vi "MainVI_Project3.vi"() -> ()   [LabVIEW 2025]
uses:
  <vilib>/MakerHub/LINX/Public/Peripherals/Digital/Digital Write 1 Chan.vi
  <vilib>/MakerHub/LINX/Public/Peripherals/Digital/Digital Write N Chans.vi
  <vilib>/MakerHub/LINX/Private/Local IO/LinxDigitalWrite.vi
  <vilib>/MakerHub/LINX/Public/Utilities/Check Channel.vi
  <vilib>/MakerHub/LINX/Public/Utilities/Open Serial.vi
  <vilib>/MakerHub/LINX/Private/Utilties/Generate Error.vi
  <vilib>/MakerHub/LINX/LMH-LINX.lvlib
panel:
  out "Patient's Heart Rate (BPM)":dbl format="%#_12g"
  out "Raw Signal with Smoothed Signal Waveform Graph":waveform(dbl)[](graph)
  in  "Sampling Frequency (Hz)":dbl
  in  "Sampling Duration (s)":dbl
  out "STD dt":dbl
  out "Holding Last Good HR":bool
  out "Good Signal !!":bool
  out "Full AutoCorrelation Waveform Graph":dbl[](graph)
  out "Peak Markers XY Graph":T1(graph)
  out "# Valid Peaks":i32
  in  "AutoCorrelation Peak Ratio Threshold":dbl
  in  "AutoCorrelation Max Lag":dbl
  in  "Tolerance Fraction":dbl
  out "Periodic Signal?":bool
  out "Best Lag":dbl
  out "AutoCorr Peak Amplitudes":dbl[](array[numeric])
  out "AutoCorrelation - Right Side":dbl[](array[numeric])
  out "AutoCorrelation Peak Locations":dbl[](array[numeric])
  out "Right Side AutoCorrelation Waveform Graph":dbl[](graph)
  in  "Autocorrelation Peak Width":dbl
  in  "Autocorrelation Peak Threshold":dbl
  in  "Autocorrelation Min Lag":dbl
  in  "Max Lag Index":dbl
  in  "Min Lag Index":dbl
  out "Periods (s)":dbl[](array[numeric])
  out "Filtered Lag Array":dbl[](array[numeric])
  out "Valid HR?":bool
  out "Valid Peaks Found?":bool
  out "Peak Amplitudes":dbl[](array[numeric])
  out "Peak Locations":dbl[](array[numeric])
  in  "Peak Threshold":dbl
  in  "Peak Width":dbl
  out "Sample Count":i32
  out "Raw Voltage":dbl
  out "Heart Rate Trend Waveform Chart":dbl(graph)
  out "Heart Rate (BPM)":dbl
  out "Normalized Signal Waveform Graph":waveform(dbl)(graph)
  out "Raw Signal Waveform Graph":waveform(dbl)(graph)
  out "dt (sec)":dbl
  out "Detrended Signal Waveform Graph":waveform(dbl)(graph)
  out "Smoothed Signal Waveform Graph":waveform(dbl)(graph)
  out "Error Out":errorcluster
  in  "Serial Port":refnum<visa-resource-name>="N/A"
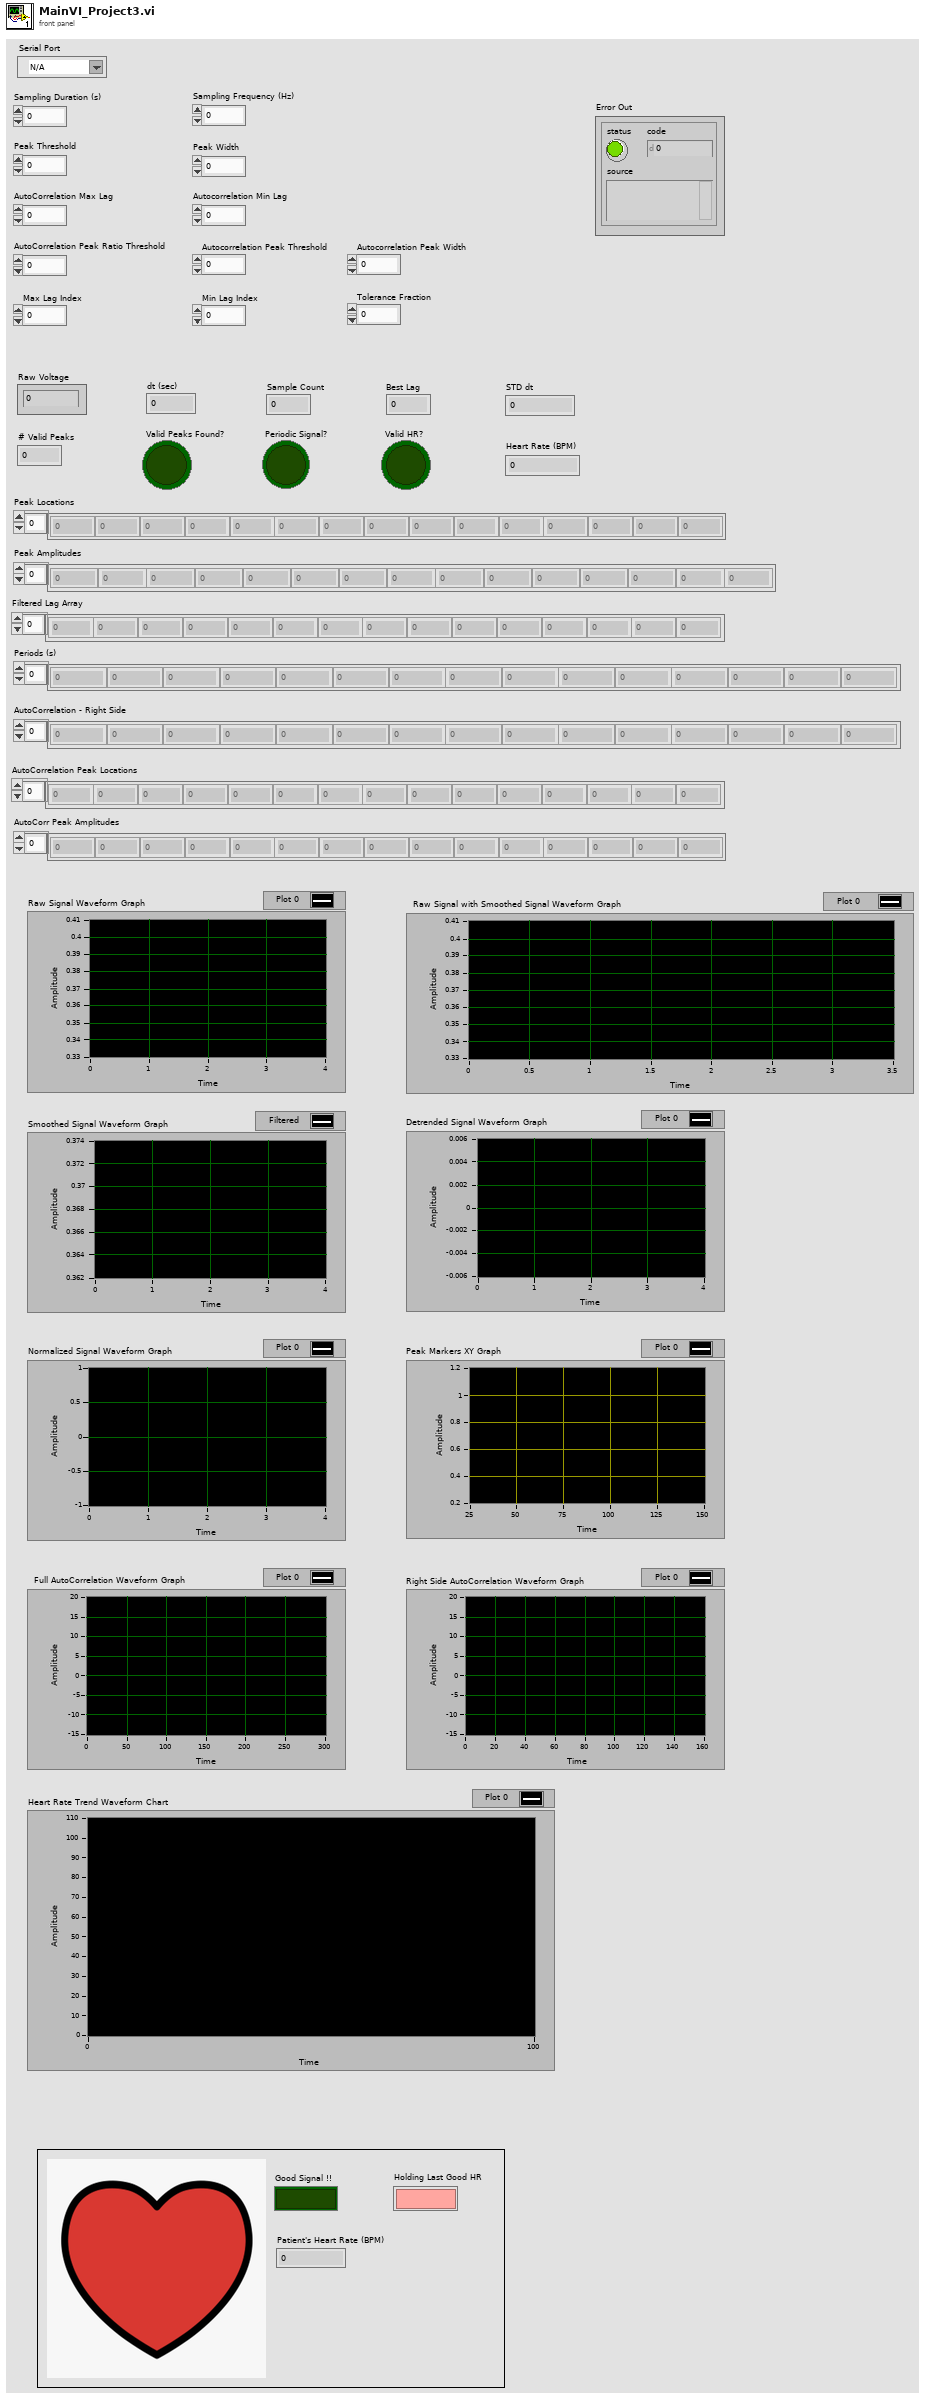
[diagram p1: front panel]
types:
  T1 = cluster{"Peak Locations":dbl[], "Peak Amplitudes":dbl[]}
  T2 = typedef "LMH-LINX.lvlib/LINX Ref.ctl" = cluster{"IO":T3, "Interface":T4, "LINX Device Config":T5}
  T3 = typedef "LMH-LINX.lvlib/Platform.ctl" = enum16{"Remote", "Local"}
  T4 = typedef "LMH-LINX.lvlib/Interface.ctl" = enum16{"Serial", "TCP"}
  T5 = typedef "LMH-LINX.lvlib/Device.lvlib/LINX Device Config.ctl" = cluster{"Interface":T4, "COM Port":refnum<visa-resource-name>, "TCP Configuration":T6, "Device Family":u8, "Device ID":u8, "Device Name":string, "TCP Ref":refnum<k5>, "Channels":T7}
  T6 = typedef "LMH-LINX.lvlib/Device.lvlib/TCP Config.ctl" = cluster{"IP Address":string, "Port":u16}
  T7 = typedef "LMH-LINX.lvlib/Channels.ctl" = cluster{"DI":u8[], "DO":u8[], "AI":u8[], "AO":u8[], "PWM":u8[], "QE":u8[], "UART":u8[], "I2C 2":u8[], "SPI":u8[], "CAN":u8[], "Servo":u8[], "AI Ref (V)":dbl, "AI Resolution (Bits)":u8, "AO Ref (V)":dbl, "AO Resolution (Bits)":u8}
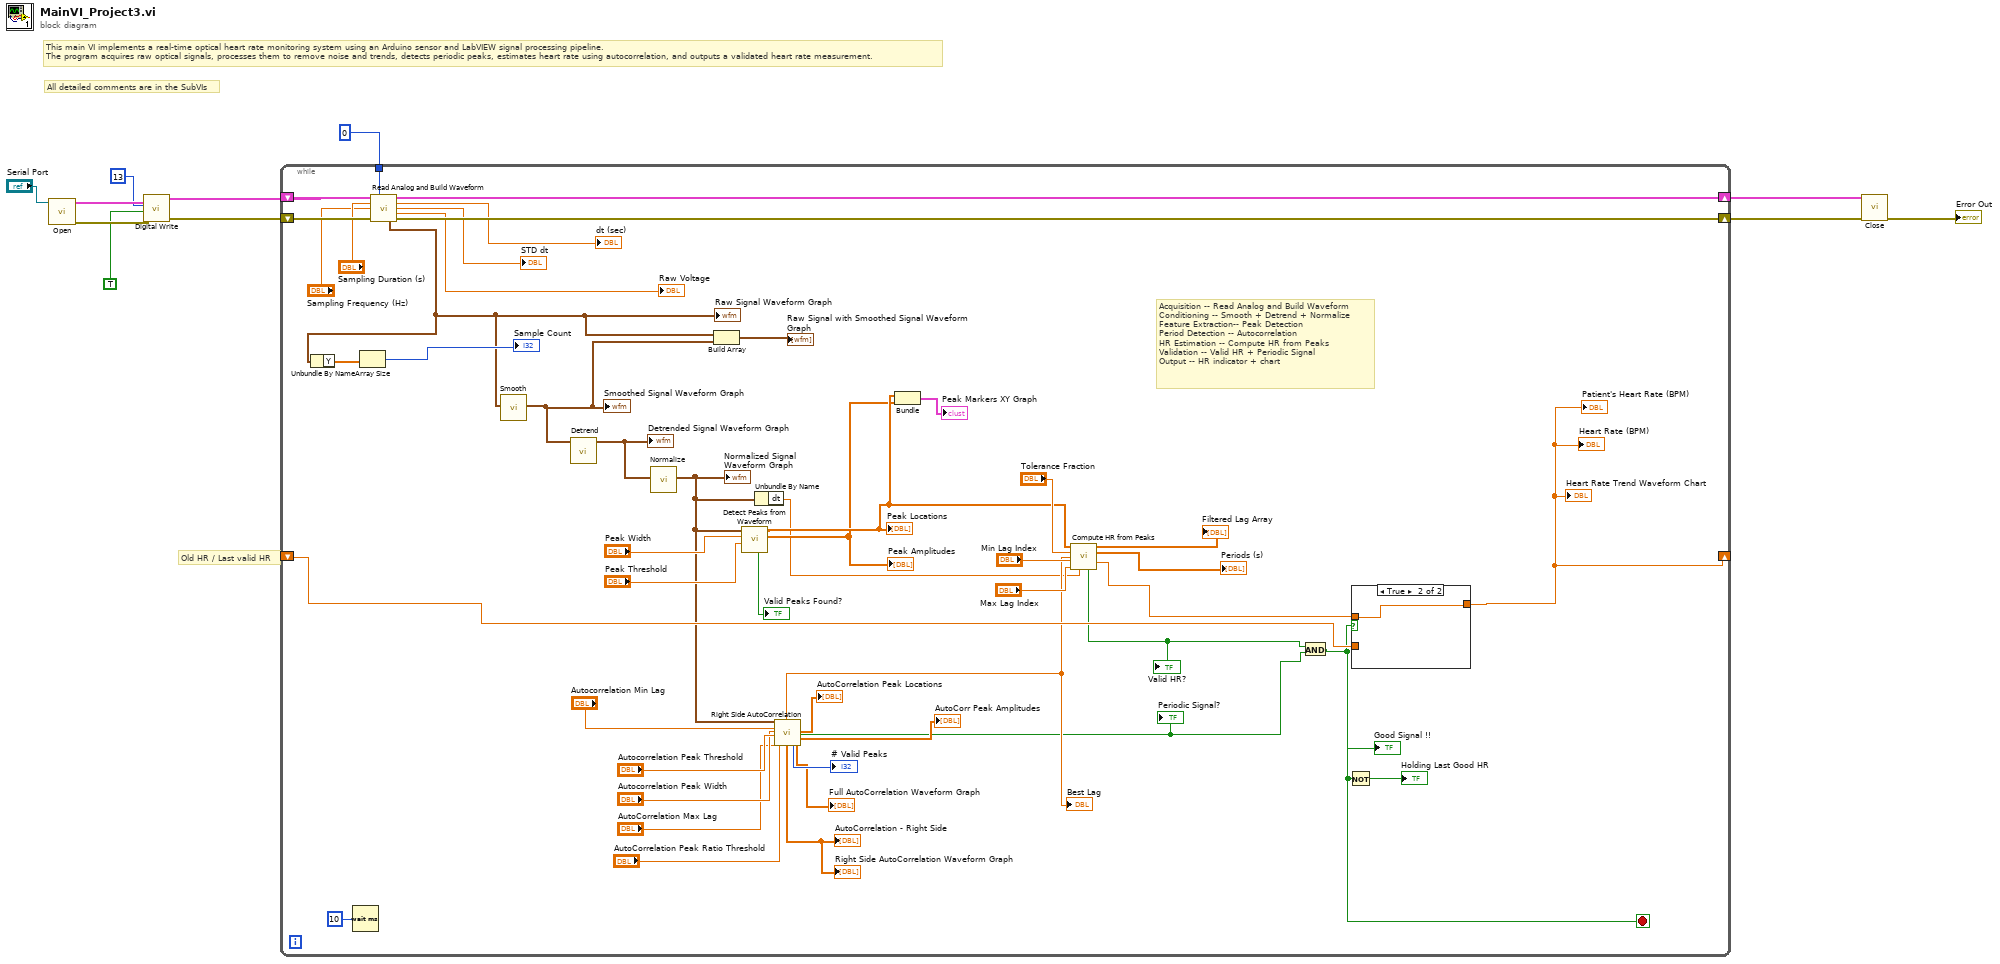
[diagram p0: block diagram]
diagram:
  # "This main VI implements a real-time optical heart rate monitoring system using an Arduino sensor and LabVIEW signal processing pipeline. \nThe program acquires raw optical signals, processes them to remove noise and trends, detects periodic peaks, estimates heart rate using autocorrelation, and outputs a validated heart rate measurement."
  # "All detailed comments are in the SubVIs"
  # "Old HR / Last valid HR"
  n1 = call-poly <vilib>:"Open.vi"("Serial Port"="Serial Port") -> ("Error Out"=w5:errorcluster, "LINX Resource"=w6:T2)  [unwired: 8 in, 1 out]
  n2 = call-poly <vilib>:"Digital Write.vi"("Error In"=w5, "Output Value"=TRUE, "DO Channel"=u8 13, "LINX Resource"=w6) -> ("Error Out"=w4:errorcluster, "LINX Resource"=w7:T2)  [unwired: 6 in]
  n3 = while {
    shift-right: [w55] -> w9
    shift-left: w7 -> [w57]
    shift-right: [w54] -> w8
    shift-left: w4 -> [w56]
    shift-right: [w12] -> _
    shift-left: _ -> [w58]
    tunnel: u8 0 ("Analog Channel") -> [w49]
    stop <- w16 stop-if-true
    # "Acquisition --\tRead Analog and Build Waveform\nConditioning --\tSmooth + Detrend + Normalize\nFeature Extraction-- Peak Detection\nPeriod Detection --\tAutocorrelation\nHR Estimation --\tCompute HR from Peaks\nValidation --\tValid HR + Periodic Signal\nOutput --\tHR indicator + chart"
    n4 = Wait (ms)(milliseconds to wait=u32 10) -> ()  [unwired: 1 out]
    n5 = call "Read Analog and Build Waveform.vi"("LINX Resource in"=w57, "Analog Channel"=w49, "Sampling Duration (s)"="Sampling Duration (s)", "Sampling Frequency (Hz)"="Sampling Frequency (Hz)", "Error In"=w56) -> ("LINX Resource out"=w55:T2, "mean dt"=→"dt (sec)":dbl, "STD dt"=→"STD dt":dbl, "Raw Voltage"=→"Raw Voltage":dbl, "Raw Signal Waveform Out"=w15:waveform(dbl), "Error Out"=w54:errorcluster)  [unwired: 5 in]
    "Raw Signal Waveform Graph" <- w15
    n6 = Unbundle By Name(w15) -> ("Y"=w48:dbl[])
    n7 = Array Size(array=w48) -> (size(s)=→"Sample Count":i32)
    n8 = call "Smooth.vi"("Raw Signal Waveform In"=w15) -> ("Smooth Signal Waveform Out"=w14:waveform(dbl))  [unwired: 9 in, 1 out]
    "Smoothed Signal Waveform Graph" <- w14
    n9 = call "Detrend.vi"("Smooth Signal Waveform In"=w14) -> ("Detrended Signal Waveform Out"=w45:waveform(dbl))  [unwired: 6 in, 4 out]
    "Detrended Signal Waveform Graph" <- w45
    n10 = call "Normalize.vi"("Detrended Signal Waveform In"=w45) -> ("Normalized Signal Waveform Out"=w20:waveform(dbl))  [unwired: 8 in, 2 out]
    "Normalized Signal Waveform Graph" <- w20
    n11 = Build Array(w15, w14) -> (→"Raw Signal with Smoothed Signal Waveform Graph":waveform(dbl)[])
    n12 = call "Detect Peaks from Waveform.vi"("Peak Threshold"="Peak Threshold", "Peak Width"="Peak Width", "Normalized Waveform In"=w20) -> ("Peak Amplitudes"=w25:dbl[], "Peak Locations"=w26:dbl[], "Valid Peaks Found?"=→"Valid Peaks Found?":bool)  [unwired: 4 in, 2 out]
    "Peak Locations" <- w26
    "Peak Amplitudes" <- w25
    n13 = Unbundle By Name(w20) -> ("dt"=w19:dbl)
    n14 = call "Right Side AutoCorrelation.vi"("Normalized Signal Waveform In"=w20, "Autocorrelation Peak Width"="Autocorrelation Peak Width", "Autocorrelation Peak Threshold"="Autocorrelation Peak Threshold", "AutoCorrelation Min Lag"="Autocorrelation Min Lag", "AutoCorrelation Max Lag"="AutoCorrelation Max Lag", "AutoCorrelation Peak Ratio Threshold"="AutoCorrelation Peak Ratio Threshold") -> ("Best Lag"=w28:dbl, "Autocorrelation - Right Side"=→"Right Side AutoCorrelation Waveform Graph" →"AutoCorrelation - Right Side":dbl[], "# Valid Peaks"=→"# Valid Peaks":i32, "Full Autocorrelation Waveform Graph"=→"Full AutoCorrelation Waveform Graph":dbl[], "Valid AutoCorr Peak Locations"=→"AutoCorrelation Peak Locations":dbl[], "Periodic Signal?"=w17:bool, "Valid AutoCorr Peak Amplitudes"=→"AutoCorr Peak Amplitudes":dbl[])  [unwired: 6 in, 9 out]
    "Best Lag" <- w28
    "Periodic Signal?" <- w17
    n15 = Bundle("Peak Locations"=w26, "Peak Amplitudes"=w25) -> (→"Peak Markers XY Graph":T1)  [unwired: 1 in]
    n16 = call "Compute HR from Peaks.vi"("Peak Locations In"=w26, "Tolerance Fraction"="Tolerance Fraction", "Reference Lag from AutoCorrelation"=w28, "Min Lag Index"="Min Lag Index", "Max Lag Index"="Max Lag Index", "dt"=w19) -> ("Filtered Lag Arrray"=→"Filtered Lag Array":dbl[], "Periods (s)"=→"Periods (s)":dbl[], "HR (bpm)"=w40:dbl, "valid HR?"=w18:bool)  [unwired: 2 in, 4 out]
    "Valid HR?" <- w18
    n17 = And(x=w18, y=w17) -> (x .and. y?=w16:bool)
    "Good Signal !!" <- w16
    n18 = Not(x=w16) -> (.not. x?=→"Holding Last Good HR":bool)
    n19 = case shown="True" w16 {
      tunnel: w40 -> [_ w61]
      tunnel: [w60 w61] -> w12
      tunnel: w58 -> [w60 _]
      frame False {
      }
      frame True {
      }
    }
    "Heart Rate (BPM)" <- w12
    "Heart Rate Trend Waveform Chart" <- w12
    "Patient's Heart Rate (BPM)" <- w12
  }
  n20 = call <vilib>:"Close.vi"("Error In"=w8, "LINX Resource"=w9) -> ("Error Out"=→"Error Out":errorcluster)  [unwired: 9 in]
